vi "Histogram Bin Size Definition Dialog.vi"(0 "Enable":bool=TRUE, 5 "error in (no error)":errorcluster) -> (17 "Bin":dbl format="%#g", 18 "OK":bool, 19 "error out":errorcluster)   [LabVIEW 2019, in "Histogram Window.lvlib"]
doc: "Displays a standard dialog box that prompts users to enter information, such as a user name and password.\n--------------------\n\nThis Express VI is configured as follows:\n\nMessage to Display to the User:Histogram bin to use:\nThe inputs are: \nNumber: Bin"
uses:
  Histogram Window.lvlib
panel:
  in  "Cancel":bool
  in  "Bin Size":dbl=1.0
  in  "OK":bool caption="OK1"
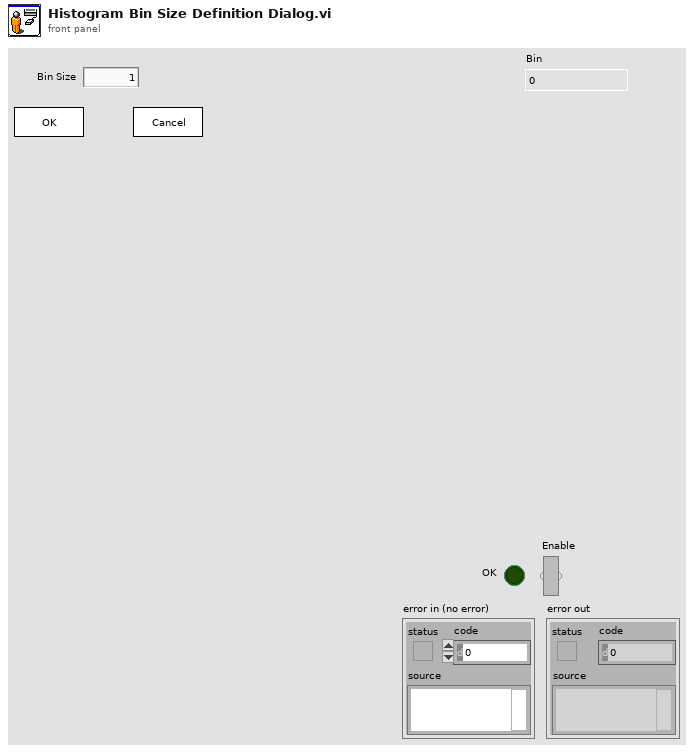
[diagram p1: front panel]
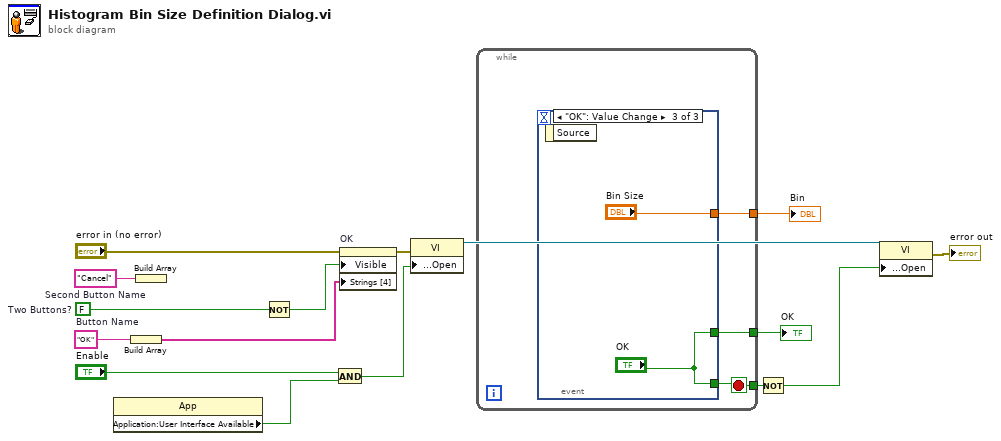
[diagram p0: block diagram]
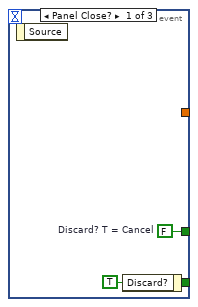
[diagram p2: hidden frame]
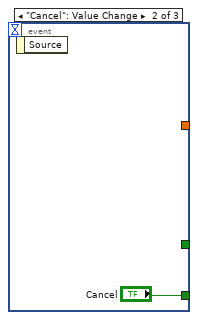
[diagram p3: hidden frame]
diagram:
  w14 = "Cancel"  # Second Button Name
  w12 = "OK"  # Button Name
  w16 = FALSE  # Two Buttons?
  n1 = property class="App"() -> ("Application:User Interface Available"=w7:bool)  [unwired: 2 in, 2 out]
  n2 = Build Array(w12) -> (w13:string[])
  n3 = Build Array(w14) -> ()  [unwired: 1 out]
  n4 = Not(x=w16) -> (.not. x?=w15:bool)
  n5 = And(x="Enable", y=w7) -> (x .and. y?=w4:bool)
  n6 = property on="OK" class="Bool"(error in="error in (no error)", "Visible"=w15, "Strings [4]"=w13) -> (error out=w11:errorcluster)  [unwired: 1 in, 1 out]
  n7 = property class="VI"(error in=w11, "Front Panel Window:Open"=w4) -> (reference out=w3:refnum<vi>)  [unwired: 1 in, 1 out]
  n8 = while {
    tunnel: [w19] -> w5
    tunnel: [w17] -> w6
    tunnel: [w18] -> w2
    stop <- w18 stop-if-true
    n9 = event shown="[2] \"OK\": Value Change" {
      selector: _ -> [_ _ _]
      dyn-events: _ -> [_ _ _]
      timeout: _ -> [_ _ _]
      tunnel: [w21 "Cancel" "OK"] -> w18
      tunnel: [w20 _ "OK"] -> w19
      tunnel: [_ _ "Bin Size"] -> w17
      event Panel Close? {
        w20 = FALSE  # Discard? T = Cancel
        w21 = TRUE ("Discard?")
        n10 = event-data() -> ()  [unwired: 1 in, 1 out]
        n11 = event-data("Discard?"=w21) -> ()  [unwired: 1 in, 1 out]
      }
      event "Cancel": Value Change {
        n12 = event-data() -> ()  [unwired: 1 in, 1 out]
      }
      event "OK": Value Change {
        n13 = event-data() -> ()  [unwired: 1 in, 1 out]
      }
    }
  }
  "OK" <- w5
  "Bin" <- w6
  n14 = Not(x=w2) -> (.not. x?=w1:bool)
  n15 = property class="VI"(reference=w3, "Front Panel Window:Open"=w1) -> (error out=→"error out":errorcluster)  [unwired: 1 in, 1 out]
